vi "TestRFGVRequestManagment.vi"() -> (0 "error out":errorcluster, 2 "Pass":bool)   [LabVIEW 2015]
uses:
  TypeDef/RequestActionEnum.ctl
  LVClasses/Request/PersonnelType.ctl
  LVClasses/Request/JsonCluster.ctl
  LVClasses/Request/Request.lvclass
panel:
  out "Added":bool
  out "Removed?":bool
  out "DataInit PUIDs":string
  out "Add Personnel 2":string
  out "Read PUIDs 2":string
  out "Remove Personnel":string
  out "Add Request":string
  out "Read Requests":string
  in  "RUID":string="r1"
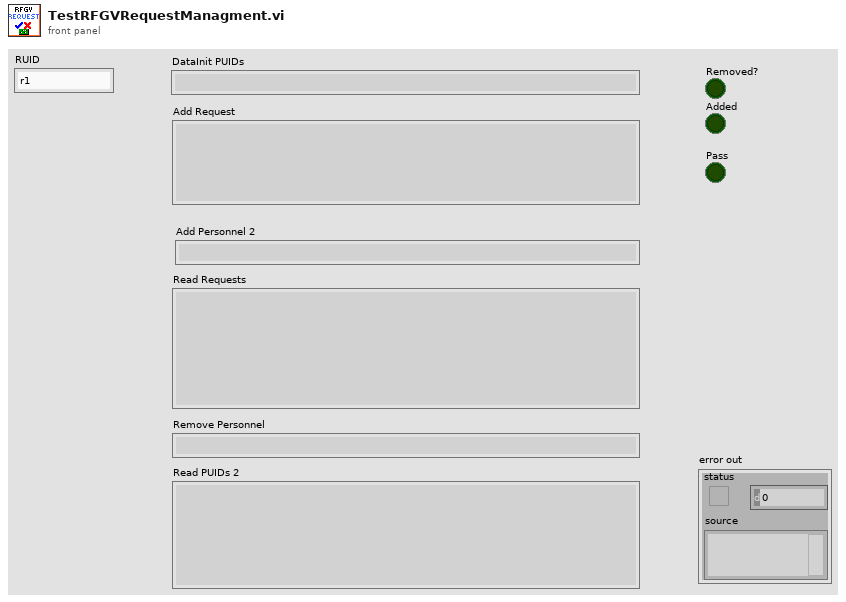
[diagram p1: front panel]
types:
  T1 = typedef "RequestActionEnum.ctl" = enum16{"Init", "ReadRequests", "ReadRequest", "AddRequest", "RemoveRequest", "ToDisk", "Ack", "Complete", "Read Summary"}
  T2 = typedef "Request.lvclass/JsonCluster.ctl" = cluster{"RequestID":string, "PersonnelType":i32, "StartTime":string, "StartName":string, "AckTime":string, "AckName":string, "FulfilledTime":string, "FulfilledName":string, "Description":string, "RoomNumber":i32, "RequestType":i32, "Alarm":bool}
  T3 = typedef "Request.lvclass/PersonnelType.ctl" = enum16{"Nurse", "Doctor", "Cleanning", "Admin"}
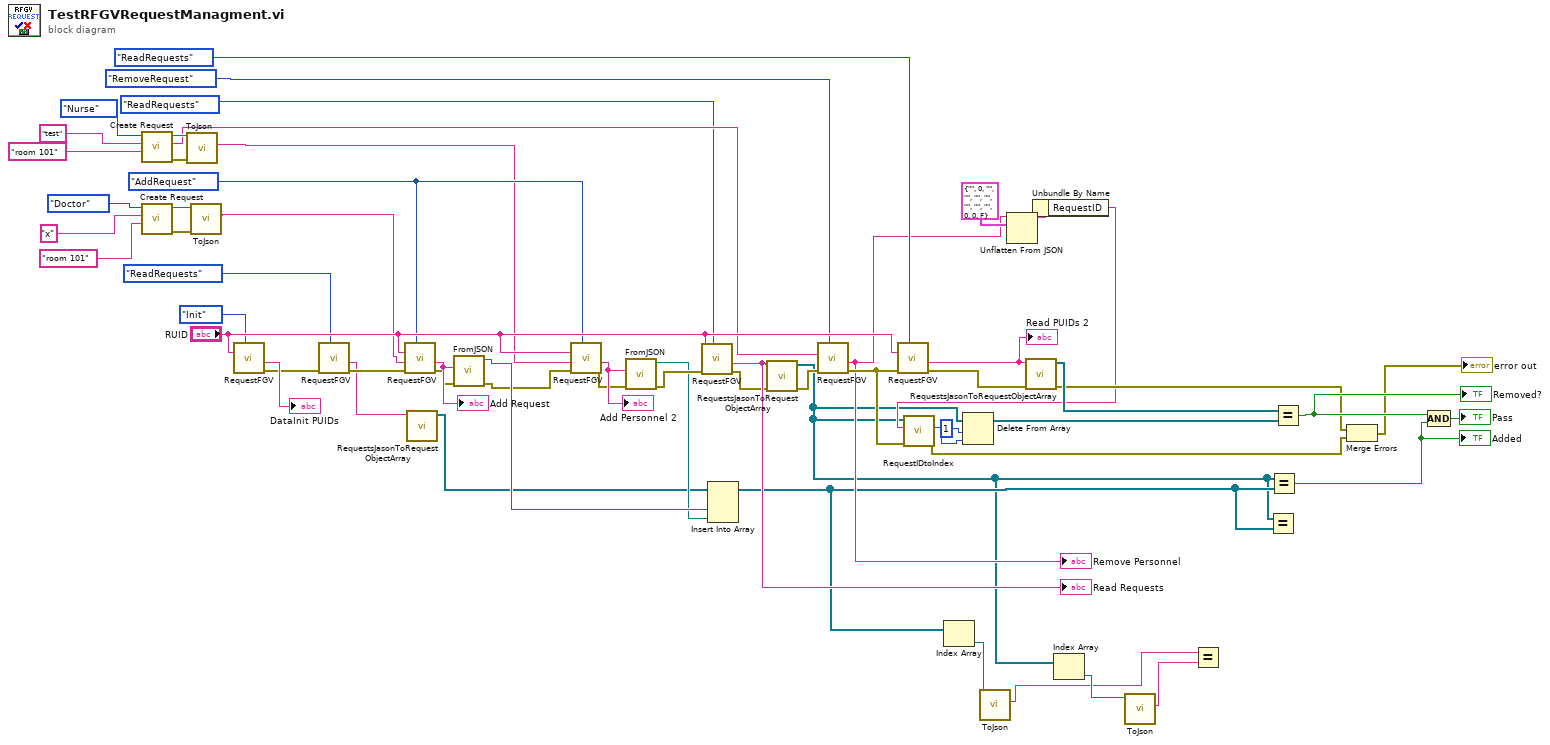
[diagram p0: block diagram]
diagram:
  w52 = RequestActionEnum."AddRequest" ("Actions")
  n1 = call "Create Request.vi"(".Description"="room 101", "Name"="test", "Personnel Type"=PersonnelType."Nurse" ("Type")) -> ("error out"=w47:errorcluster, "RUID"=w45:string, "Request out"=w51:refnum<class "Request.lvclass">)  [unwired: 6 in]
  n2 = call "Create Request.vi"(".Description"="room 101" (".Description 2"), "Name"="x" ("Name 2"), "Personnel Type"=PersonnelType."Doctor" ("Type 2")) -> ("error out"=w49:errorcluster, "Request out"=w48:refnum<class "Request.lvclass">)  [unwired: 6 in, 1 out]
  n3 = call "ToJson.vi"("error in (no error)"=w47, "Request"=w51) -> ("Request"=w50:string)  [unwired: 8 in, 1 out]
  n4 = call "ToJson.vi"("error in (no error)"=w49, "Request"=w48) -> ("Request"=w46:string)  [unwired: 8 in, 1 out]
  n5 = call "RequestFGV.vi"("Actions"=RequestActionEnum."Init", "RUID"="RUID") -> ("error out"=w35:errorcluster, "Data Out"=→"DataInit PUIDs":string)  [unwired: 8 in]
  n6 = call "RequestFGV.vi"("Actions"=RequestActionEnum."ReadRequests", "error in (no error)"=w35) -> ("error out"=w10:errorcluster, "Data Out"=w8:string)  [unwired: 8 in]
  n7 = call "RequestFGV.vi"("Actions"=w52, "error in (no error)"=w10, "Data In"=w46, "RUID"="RUID") -> ("error out"=w28:errorcluster, "Data Out"=w34:string)  [unwired: 6 in]
  "Add Request" <- w34
  n8 = call "RequestsJasonToRequestObjectArray.vi"("Requests"=w8) -> ("REquests"=w7:refnum<class "Request.lvclass">[])  [unwired: 9 in, 1 out]
  n9 = call "FromJSON.vi"("error in (no error)"=w28, "Request"=w34) -> ("error out"=w29:errorcluster, "Request out"=w33:refnum<class "Request.lvclass">)  [unwired: 8 in]
  n10 = call "RequestFGV.vi"("Actions"=w52, "error in (no error)"=w29, "Data In"=w50, "RUID"="RUID") -> ("error out"=w30:errorcluster, "Data Out"=w32:string)  [unwired: 6 in]
  "Add Personnel 2" <- w32
  n11 = call "FromJSON.vi"("error in (no error)"=w30, "Request"=w32) -> ("error out"=w31:errorcluster, "Request out"=w27:refnum<class "Request.lvclass">)  [unwired: 8 in]
  n12 = call "RequestFGV.vi"("Actions"=RequestActionEnum."ReadRequests", "error in (no error)"=w31, "RUID"="RUID") -> ("error out"=w24:errorcluster, "Data Out"=w26:string)  [unwired: 7 in]
  "Read Requests" <- w26
  n13 = Insert Into Array(array=w7, new element #1=w33, new element #2=w27) -> (w6:refnum<class "Request.lvclass">[])  [unwired: 1 in]
  n14 = call "RequestsJasonToRequestObjectArray.vi"("error in (no error)"=w24, "Requests"=w26) -> ("error out"=w25:errorcluster, "REquests"=w5:refnum<class "Request.lvclass">[])  [unwired: 8 in]
  n15 = call "RequestFGV.vi"("Actions"=RequestActionEnum."RemoveRequest", "error in (no error)"=w25, "RUID"=w45) -> ("error out"=w18:errorcluster, "Data Out"=w13:string)  [unwired: 7 in]
  "Remove Personnel" <- w13
  n16 = call "RequestFGV.vi"("Actions"=RequestActionEnum."ReadRequests", "error in (no error)"=w18, "RUID"="RUID") -> ("error out"=w21:errorcluster, "Data Out"=w20:string)  [unwired: 7 in]
  "Read PUIDs 2" <- w20
  n17 = Index Array(array=w6) -> (element=w4:refnum<class "Request.lvclass">)  [unwired: 1 in]
  n18 = call "ToJson.vi"("Request"=w4) -> ("Request"=w1:string)  [unwired: 9 in, 1 out]
  n19 = Unflatten From JSON(JSON string=w13, type and defaults=T2 {"RequestID"="", "PersonnelType"=0, "StartTime"="", "StartName"="", "AckTime"="", "AckName"="", "FulfilledTime"="", "FulfilledName"="", "Description"="", "RoomNumber"=0, "RequestType"=0, "Alarm"=FALSE} ("RequestTable")) -> (value=w12:T2)  [unwired: 5 in, 1 out]
  n20 = call "RequestsJasonToRequestObjectArray.vi"("error in (no error)"=w21, "Requests"=w20) -> ("error out"=w16:errorcluster, "REquests"=w19:refnum<class "Request.lvclass">[])  [unwired: 8 in]
  n21 = Unbundle By Name(w12) -> ("RequestID"=w11:string)
  n22 = call "RequestIDtoIndex.vi"("error in (no error)"=w18, "RUID"=w11, "REquest In"=w5) -> ("error out"=w17:errorcluster, "Index"=w23:i32)  [unwired: 5 in, 2 out]
  n23 = Delete From Array(array=w5, length=1, index=w23) -> (array with subset deleted=w22:refnum<class "Request.lvclass">[])  [unwired: 1 out]
  n24 = Index Array(array=w5) -> (element=w3:refnum<class "Request.lvclass">)  [unwired: 1 in]
  n25 = call "ToJson.vi"("Request"=w3) -> ("Request"=w2:string)  [unwired: 9 in, 1 out]
  n26 = Equal?(x=w1, y=w2) -> ()  [unwired: 1 out]
  n27 = Equal?(x=w5, y=w6) -> ()  [unwired: 1 out]
  n28 = Equal?(x=w5, y=w6) -> (x = y?=w57:bool)
  "Added" <- w57
  n29 = Equal?(x=w19, y=w22) -> (x = y?=w59:bool)
  "Removed?" <- w59
  n30 = Merge Errors(w16, w17) -> (→"error out":errorcluster)
  n31 = Compound Arithmetic op=AND(w59, w57) -> (→"Pass":bool)
